vi "Test_Compute_Text_Size.vi"(8 "error in (no error)":errorcluster, 11 "Test Case In":refnum<class "Image.lvclass">) -> (0 "error out":errorcluster, 3 "Test Case Out":refnum<class "Image.lvclass">)   [LabVIEW 2020, in "g_ar_toolkit.test.lvlib" / "Image.lvclass"]
uses:
  Image.lvclass
  Image.lvclass/Image.ctl
  g_ar_toolkit.image/Font Face.ctl
  g_ar_toolkit.image/g_ar_toolkit.image.lvlib
  g_ar_toolkit.image/Text Drawing Settings.ctl
  g_ar_toolkit.image/Image Size (Fixed).ctl
  4993e8ee-a06a-463a-9684-69129f64d5ce.vi
panel:
  out "Size":T1
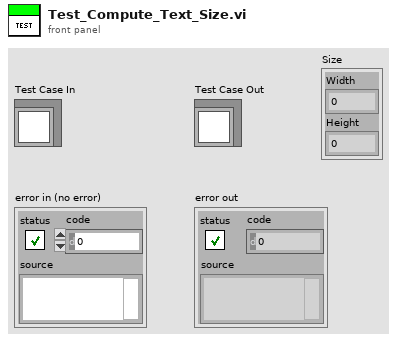
[diagram p1: front panel]
types:
  T1 = typedef "g_ar_toolkit.image.lvlib/Image Size (Fixed).ctl" = cluster{"Width":u16, "Height":u16}
  T2 = typedef "g_ar_toolkit.image.lvlib/Text Drawing Settings.ctl" = cluster{"OpenCV Font Face":T3, "Font Scale":dbl}
  T3 = typedef "g_ar_toolkit.image.lvlib/Font Face.ctl" = enum16{"FONT_HERSHEY_SIMPLEX", "FONT_HERSHEY_PLAIN", "FONT_HERSHEY_DUPLEX", "FONT_HERSHEY_COMPLEX", "FONT_HERSHEY_TRIPLEX", "FONT_HERSHEY_COMPLEX_SMALL", "FONT_HERSHEY_SCRIPT_SIMPLEX", "FONT_HERSHEY_SCRIPT_COMPLEX", "FONT_ITALIC"}
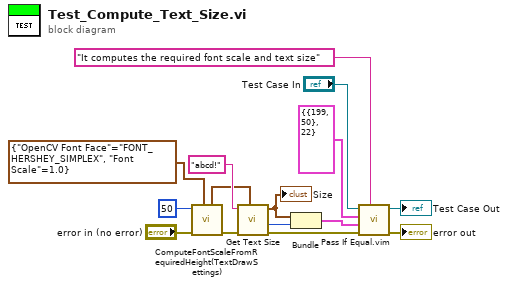
[diagram p0: block diagram]
diagram:
  n1 = call "ComputeFontScaleFromRequiredHeight(TextDrawSettings).vi"("Text Drawing Settings in (Default: Simplex)"=T2 {"OpenCV Font Face"=enum."FONT_HERSHEY_SIMPLEX", "Font Scale"=1.0} ("Text Drawing Settings (Default: Simplex, Top-Left)"), "error in (no error)"="error in (no error)", "Required Text Height"=u16 50) -> ("error out"=w10:errorcluster, "Text Drawing Settings out"=w7:T2)  [unwired: 7 in]
  n2 = call "Get Text Size.vi"("Text Drawing Settings (Default: Simplex)"=w7, "error in (no error)"=w10, "Text"="abcd!") -> ("error out"=w5:errorcluster, "Base Line"=w3:i32, "Size"=w4:T1)  [unwired: 6 in]
  "Size" <- w4
  n3 = Bundle("Size"=w4, "Base Line"=w3) -> (w2:cluster{"Size":T1, "Base Line":i32})  [unwired: 1 in]
  n4 = call "Pass If Equal.vim"("Description"="It computes the required font scale and text size", "error in (no error)"=w5, "Actual"=w2, "Expected"=cluster{"Size":T1, "Base Line":i32} {"Size"={"Width"=199, "Height"=50}, "Base Line"=22}, "LUnit Test Case In"="Test Case In") -> ("error out"=→"error out":errorcluster, "LUnit Test Case Out"=→"Test Case Out":refnum<class "Image.lvclass">)  [unwired: 5 in]
